vi "Error Dialog.vi"(8 "error in":errorcluster, 11 "FP Controls":refnum<class "FP Controls.lvclass">) -> (0 "error out":errorcluster)   [LabVIEW 2012, in "Configuration Grandmaster.lvlib" / "FP Controls.lvclass"]
uses:
  FP Controls.lvclass
  FP Controls.lvclass/FP Controls.ctl
  <vilib>/Utility/error.llb/DialogType.ctl
panel:
  out "status":bool
  out "Description":string
  out "ErrTimeStr":string
  out "Code":i32
  in  "ErrOK":bool
  # "Error Date/Time"
  # "Error Code"
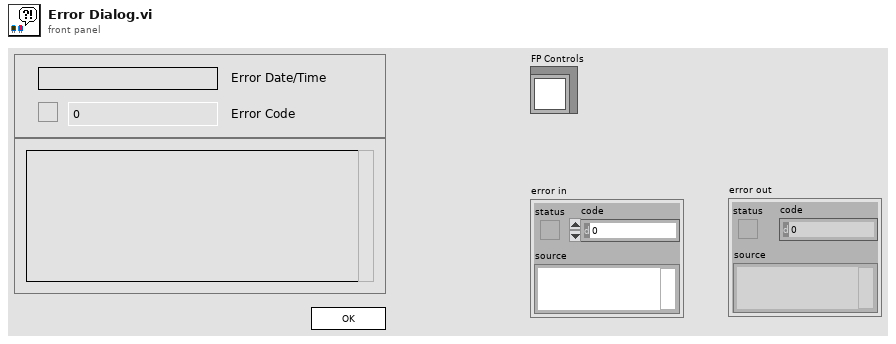
[diagram p1: front panel]
types:
  T1 = typedef "DialogType.ctl" = u16
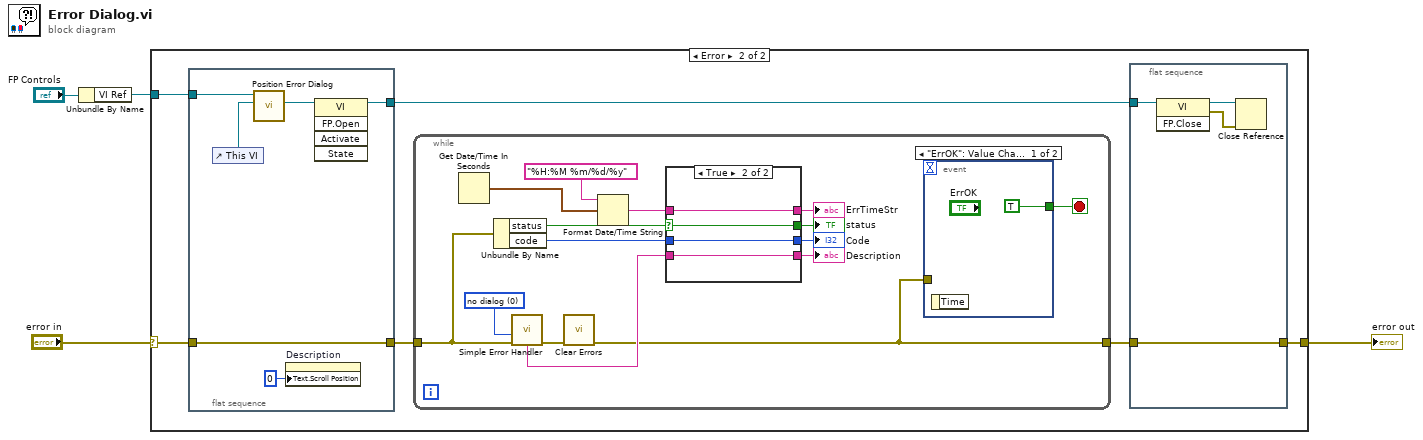
[diagram p0: block diagram]
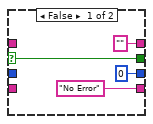
[diagram p3: hidden frame]
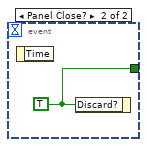
[diagram p4: hidden frame]
diagram:
  n1 = Unbundle By Name("FP Controls") -> ("VI Ref"=w1:refnum<vi>)
  n2 = case shown="Error" "error in" {
    selector: "error in" -> [w5 w11]
    tunnel: [w5 w6] -> w3
    tunnel: w1 -> [_ w9]
    frame No Error {
    }
    frame Error {
      n3 = flat-sequence {
        tunnel: w11 -> [w20]
        tunnel: [w20] -> w10
        tunnel: w9 -> [w19]
        tunnel: [w18] -> w8
        frame #0 {
          n4 = control-ref of="This VI"() -> (w17:refnum<vi>)
          n5 = call "Position Error Dialog.vi"("Err Dialog Ref"=w17, "DAQMan Ref"=w19) -> ("Dialog Ref Out"=w16:refnum<vi>)  [unwired: 9 in]
          n6 = property on="Description" class="Str"("Text.Scroll Position"=u32 0) -> ()  [unwired: 2 in, 2 out]
          n7 = invoke class="VI" method="FP.Open"(reference=w16) -> (reference out=w18:refnum<vi>)  [unwired: 4 in, 4 out]
        }
      }
      n8 = while {
        tunnel: w10 -> [w26]
        tunnel: [w22] -> w7
        stop <- w24 stop-if-true
        w28 = T1 0 items=["no dialog", "OK message", "continue or stop message", "OK message + warnings", "continue/stop + warnings"] ("type of dialog (OK msg:1)")
        n9 = Get Date/Time In Seconds() -> (seconds since 1Jan1904=w25:timestamp)
        n10 = Unbundle By Name(w26) -> ("status"=w35:bool, "code"=w33:i32)
        n11 = call <vilib>:"Simple Error Handler.vi"("type of dialog (OK msg:1)"=w28, "error in (no error)"=w26) -> ("error out"=w23:errorcluster, "message"=w27:string)  [unwired: 3 in, 3 out]
        n12 = call <vilib>:"Clear Errors.vi"("error in (no error)"=w23) -> ("error out"=w22:errorcluster)  [unwired: 6 in]
        n13 = Format Date/Time String(time format string (%c)="%H:%M %m/%d/%y", seconds (now)=w25) -> (date/time string=w34:string)  [unwired: 1 in]
        n14 = case shown="True" w35 {
          selector: w35 -> [w40 w44]
          tunnel: [w40 w44] -> w29
          tunnel: w34 -> [_ w43]
          tunnel: w33 -> [_ w42]
          tunnel: ["" ("date/time string") w43] -> w32
          tunnel: [0 ("code") w42] -> w31
          tunnel: ["No Error" ("source") w41] -> w30
          tunnel: w27 -> [_ w41]
          frame False {
          }
          frame True {
          }
        }
        "ErrTimeStr" <- w32
        "Code" <- w31
        "Description" <- w30
        "status" <- w29
        n15 = event shown="[0] \"ErrOK\": Value Change" {
          selector: _ -> [_ _]
          dyn-events: _ -> [_ _]
          timeout: _ -> [_ _]
          tunnel: [TRUE ("Discard?") w46] -> w24
          tunnel: w22 -> [_ _]
          event "ErrOK": Value Change {
            n16 = event-data() -> ()  [unwired: 1 in, 1 out]
          }
          event Panel Close? {
            w46 = TRUE ("Discard?")
            n17 = event-data() -> ()  [unwired: 1 in, 1 out]
            n18 = event-data("Discard?"=w46) -> ()  [unwired: 1 in, 1 out]
          }
        }
      }
      n19 = flat-sequence {
        tunnel: w8 -> [w15]
        tunnel: w7 -> [w14]
        tunnel: [w14] -> w6
        frame #0 {
          n20 = invoke class="VI" method="FP.Close"(reference=w15) -> (reference out=w12:refnum<vi>, error out=w13:errorcluster)  [unwired: 2 in, 1 out]
          n21 = Close Reference(reference=w12, error in (no error)=w13) -> ()  [unwired: 1 out]
        }
      }
    }
  }
  "error out" <- w3
